vi "get error string from code.vi"(8 "error in (no error)":errorcluster, 11 "errnum":i32) -> (0 "error out":errorcluster, 3 "function return":string)   [LabVIEW 2013, in "lvnano.lvlib"]
doc: "NN_EXPORT const char *nn_strerror (int errnum);"
uses:
  lvnano.lvlib
  lvnanomsg.dll
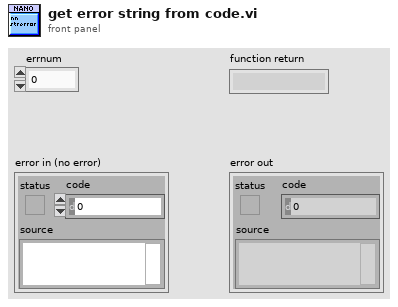
[diagram p1: front panel]
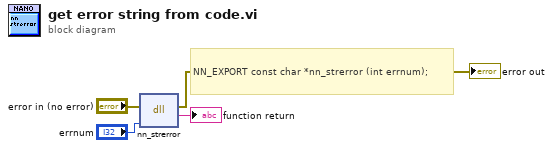
[diagram p0: block diagram]
diagram:
  # "NN_EXPORT const char *nn_strerror (int errnum);"
  n1 = dll-call lib="C:/Users/Daniel/Documents/nanomsg/lvnano/lvnanomsg.*" fn="nn_strerror"(error in="error in (no error)", "errnum"="errnum") -> (error out=→"error out":errorcluster, →"function return":string)  [unwired: 3 in, 1 out]
